vi "Event Self.vi"(10 "Msg Strategy":refnum<class "Msg Strategy.lvclass">, 11 "Base Event jettl in":refnum<class "Base Event jettl.lvclass">) -> (3 "Base Event jettl out":refnum<class "Base Event jettl.lvclass">)   [LabVIEW 2021, in "jettl.lvlib" / "Base Event jettl.lvlib" / "Base Event jettl.lvclass"]
uses:
  Base Event jettl.lvclass
  Msg Strategy/Msg Strategy.lvclass
  Base Event jettl.lvclass/Base Event jettl.ctl
  jettl.lvlib
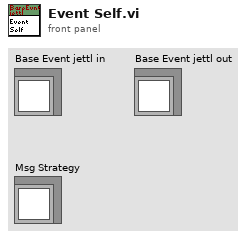
[diagram p1: front panel]
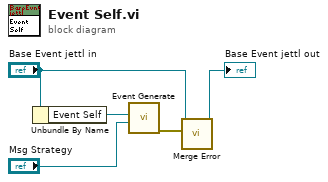
[diagram p0: block diagram]
diagram:
  n1 = Unbundle By Name("Base Event jettl in") -> ("Event Self"=w1:refnum<data-value>)
  n2 = call "Event Generate.vi"("Msg Strategy"="Msg Strategy", "Event"=w1) -> ("error out"=w3:errorcluster)  [unwired: 9 in]
  n3 = call-dynamic "Merge Error.vi"("Error"=w3, "Base Event jettl in"="Base Event jettl in") -> ("Base Event jettl out"=→"Base Event jettl out":refnum<class "Base Event jettl.lvclass">)  [unwired: 9 in]
